vi "OM_FromLabVIEW.vi"(8 "error in (no error)":errorcluster, 11 "ObjectLUT in":refnum<class "ObjectLUT.lvclass">) -> (0 "error out":errorcluster, 2 "DbRow":variant, 3 "ObjectLUT out":refnum<class "ObjectLUT.lvclass">)   [LabVIEW 2020, in "ORM_lib.lvlib" / "ObjectLUT.lvclass"]
uses:
  ObjectLUT.lvclass
  ObjectLUT.lvclass/ObjectLUT.ctl
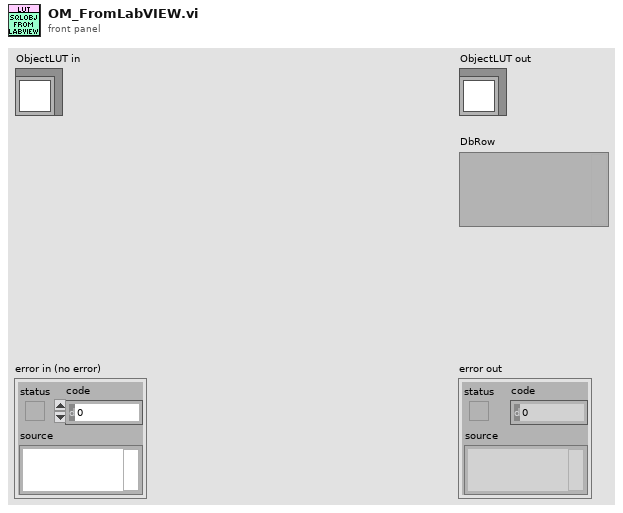
[diagram p1: front panel]
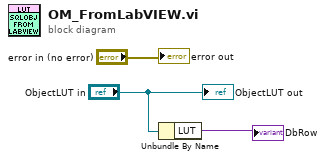
[diagram p0: block diagram]
diagram:
  n1 = Unbundle By Name("ObjectLUT in") -> ("LUT"=→"DbRow":variant)
  "error out" <- "error in (no error)"
  "ObjectLUT out" <- "ObjectLUT in"
